vi "GetPVUnitsChar.vi"(8 "error in":errorcluster, 10 "Channel number":i32, 11 "VISA resource name":refnum<visa-resource-name>) -> (0 "error out":errorcluster, 2 "ascii units character":string, 3 "VISA resource name out":refnum<visa-resource-name>)   [LabVIEW 2023, in "Thermotron 8800.lvlib"]
doc: "CCHR\nCommand name: Send process variable units character\nCommand type: System status\nDescription: The 8800 returns the ASCII units for the character. Common unit codes are C (Celsius),\nF (Fahrenheit), % (percent relative humidity), and T (torr).\nSyntax: CCHRn?\nWhere n is any process variable channel (1 to 8) or monitor channel (9-16).\nNOTE: 9 = monitor channel 1, 10 = monitor channel 2, etc.\nData type: ASCII units character\nQuery example: CCHR1?\n8800 response: C (Channel 1 is programmed in degrees Celsius.)"
uses:
  Thermotron 8800.lvlib
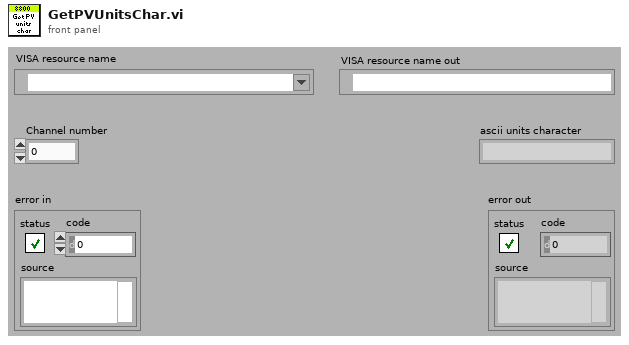
[diagram p1: front panel]
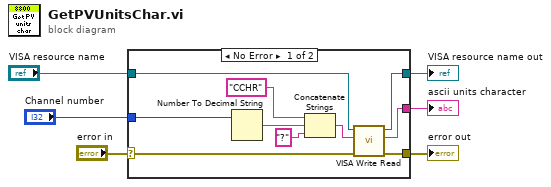
[diagram p0: block diagram]
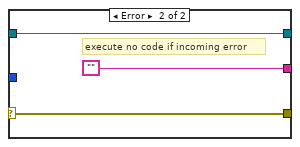
[diagram p2: hidden frame]
diagram:
  n1 = case shown="No Error" "error in" {
    selector: "error in" -> [w10 w18]
    tunnel: "Channel number" -> [w12 _]
    tunnel: "VISA resource name" -> [w11 w19]
    tunnel: [w9 w18] -> w3
    tunnel: [w8 ""] -> w2
    tunnel: [w7 w19] -> w1
    frame No Error {
      n2 = Number To Decimal String(number=w12) -> (decimal integer string=w15:string)  [unwired: 1 in]
      n3 = Concatenate Strings("CCHR" ("string"), w15, "?" ("string")) -> (w13:string)
      n4 = call "VISA Write Read.vi"("error in (no error)"=w10, "8800 Command"=w13, "VISA Refnum in"=w11) -> ("error out"=w9:errorcluster, "read buffer"=w8:string, "VISA Refnum out"=w7:refnum<visa-resource-name>)  [unwired: 6 in]
    }
    frame Error {
      # "execute no code if incoming error"
    }
  }
  "error out" <- w3
  "ascii units character" <- w2
  "VISA resource name out" <- w1
